vi "Rohde & Schwarz VNA Restore.vi"(7 "Rohde & Schwarz VNA":T1, 8 "error in (no error)":errorcluster, 11 "VISA Resource Name":refnum<visa-resource-name>) -> (0 "error out":errorcluster {"code" format="%.0x"}, 3 "dup VISA Resource Name":refnum<visa-resource-name>)   [LabVIEW 2011]
uses:
  TypeDefs/Rohde & Schwarz VNA Instrument Info.ctl
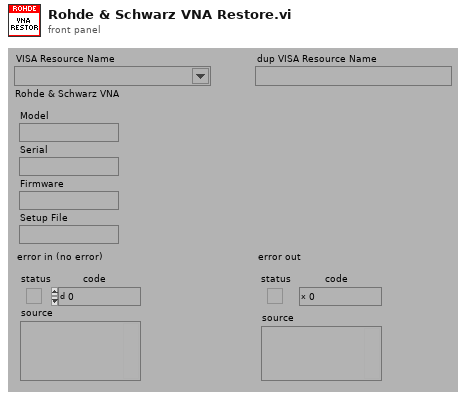
[diagram p1: front panel]
types:
  T1 = typedef "Rohde & Schwarz VNA Instrument Info.ctl" = cluster{"Model":string, "Serial":string, "Firmware":string, "Setup File":string}
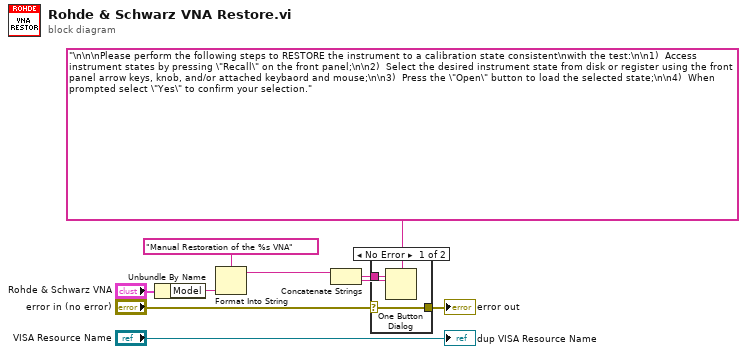
[diagram p0: block diagram]
diagram:
  n1 = Unbundle By Name("Rohde & Schwarz VNA") -> ("Model"=w7:string)
  n2 = Format Into String(format string="Manual Restoration of the %s VNA", w7) -> (resulting string=w6:string)  [unwired: 2 in, 1 out]
  n3 = Concatenate Strings(w6, "\n\n\nPlease perform the following steps to RESTORE the instrument to a calibration state consistent\nwith the test:\n\n1)  Access instrument states by pressing \"Recall\" on the front panel;\n\n2)  Select the desired instrument state from disk or register using the front panel arrow keys, knob, and/or attached keybaord and mouse;\n\n3)  Press the \"Open\" button to load the selected state;\n\n4)  When prompted select \"Yes\" to confirm your selection.") -> (w4:string)
  n4 = case shown="No Error" "error in (no error)" {
    selector: "error in (no error)" -> [w10 w12]
    tunnel: w4 -> [w11 _]
    tunnel: [w10 w12] -> w2
    frame No Error {
      n5 = One Button Dialog(message=w11) -> ()  [unwired: 2 out]
    }
    frame Error {
    }
  }
  "error out" <- w2
  "dup VISA Resource Name" <- "VISA Resource Name"
